vi "test Import Invalid Configuration Files.vi"(8 "error in":errorcluster, 11 "TestCase in":refnum<class "Import.lvclass">) -> (0 "error out":errorcluster, 3 "TestCase out":refnum<class "Import.lvclass">)   [LabVIEW 2024, in "Import.lvclass"]
uses:
  Import.lvclass
  <vilib>/addons/_JKI Toolkits/VI Tester/TestCase.llb/TestCase.lvclass
  Import/ARINC 429 Import.lvlib
  <vilib>/NI/VeriStand Custom Device Testing Tools/VeriStandTestUtilities/VeriStandTestUtilities.lvlib
  C:/Program Files/National Instruments/LabVIEW 2024/vi.lib/addons/_JKI Toolkits/VI Tester/TestCase.llb/TestCase.lvclass
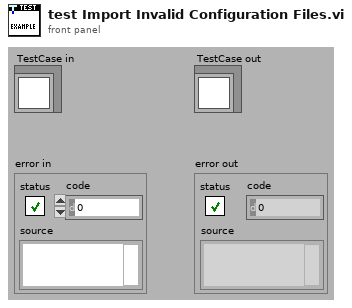
[diagram p1: front panel]
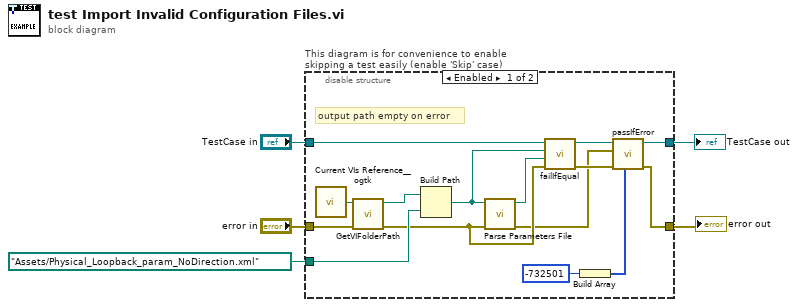
[diagram p0: block diagram]
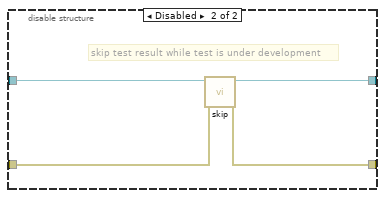
[diagram p2: hidden frame]
diagram:
  n1 = disable-structure "This diagram is for convenience to enable skipping a test easily (enable 'Skip' case)" shown="Enabled" {
    disable-tunnel: "TestCase in" -> [w20 w24]
    disable-tunnel: [w11 w22] -> w2
    disable-tunnel: [w10 w23] -> w4
    disable-tunnel: "error in" -> [w17 w21]
    disable-tunnel: path "Assets/Physical_Loopback_param_NoDirection.xml" ("Absolute or Relative Path") -> [w16 _]
    frame Enabled {
      # "output path empty on error"
      n2 = call <userlib>:"Current VIs Reference__ogtk.vi"() -> ("Current VI's reference"=w19:refnum<vi>)  [unwired: 5 in]
      n3 = call <vilib>:"GetVIFolderPath.vi"("error in (no error)"=w17, "VI Reference in"=w19) -> ("error out"=w12:errorcluster, "VI Folder Path out"=w18:path)  [unwired: 8 in]
      n4 = Build Path(base path=w18, name or relative path=w16) -> (appended path=w15:path)
      n5 = call "Parse Parameters File.vi"("error in"=w12, "path to XML document"=w15) -> ("error out"=w9:errorcluster, "path to XML document out"=w6:path)  [unwired: 7 in, 1 out]
      n6 = call-dynamic "failIfEqual.vi"("error in (no error)"=w12, "y"=w6, "x"=w15, "TestCase in"=w20) -> ("error out"=w13:errorcluster, "TestCase out"=w14:refnum<class "Import.lvclass">)  [unwired: 6 in]
      n7 = Build Array(-732501 ("code")) -> (w7:i32[])
      n8 = call-dynamic "passIfError.vi"("passing error codes (default = any error code)"=w7, "error in (no error)"=w13, "error"=w9, "TestCase in"=w14) -> ("error out"=w10:errorcluster, "TestCase out"=w11:refnum<class "Import.lvclass">)  [unwired: 6 in]
    }
    frame Disabled {
      # "skip test result while test is under development"
      n9 = call <vilib>:"skip.vi"("error in (no error)"=w21, "TestCase in"=w24) -> ("error out"=w23:errorcluster, "TestCase out"=w22:refnum<class "Import.lvclass">)  [unwired: 8 in]
    }
  }
  "error out" <- w4
  "TestCase out" <- w2
